vi "GetSetServiceRequestEventMask.vi"(0 "VISA resource name":refnum<visa-resource-name>, 5 "get/set":T1, 7 "Mask bits":u8 step=1, 11 "error in":errorcluster) -> (4 "VISA resource name out":refnum<visa-resource-name>, 6 "SRQ event mask string":string, 8 "SRQ event mask":i32, 10 "SRQ event mask binary":string, 15 "error out":errorcluster)   [LabVIEW 2023, in "Thermotron 8800.lvlib"]
doc: "SRQM\nCommand name: Send or load service request event mask byte\nCommand type: System status\nDescription: This byte enables the various events for requesting service via the GPIB SRQ line. The coded integer data represents the enabled events using the definitions given under the SRQB command.\nNOTE: Setting the SRQ mask to zero disables all SRQ interrupts.\nSyntax: SRQM? or SRQMdata\nData type: Coded integer (0 to 255)\nQuery example: SQRM?\n8800 response: 4 = 00000100 (The end of interval service request bit has been enabled.)\nbit 7 bit 6 bit 5 bit 4 bit 3 bit 2 bit 1 bit 0\n 0 0 0 0 0 1 0 0\nOperation example: SRQM1\n8800 response: 0 (The 8800 loads the SRQ mask with the value 1, enabling the state change SRQ event.)\nbit 7 bit 6 bit 5 bit 4 bit 3 bit 2 bit 1 bit 0\n 0 0 0 0 0 0 0 1"
uses:
  Thermotron 8800.lvlib
  Private/get set.ctl
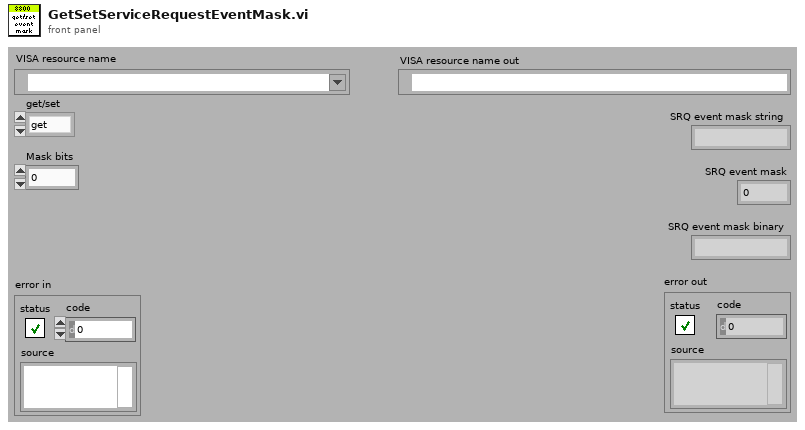
[diagram p1: front panel]
types:
  T1 = typedef "Thermotron 8800.lvlib/get set.ctl" = enum16{"get", "set"}
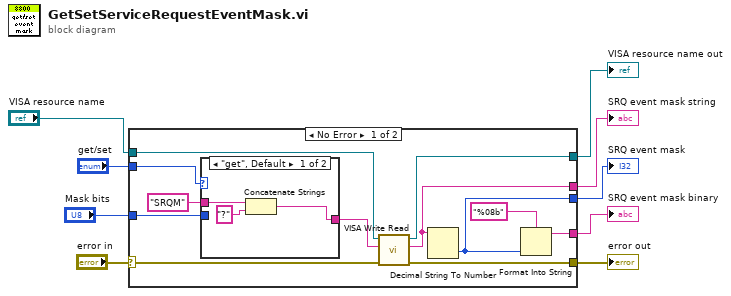
[diagram p0: block diagram]
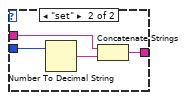
[diagram p2: hidden frame]
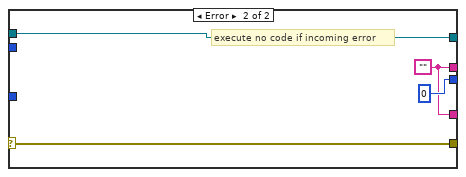
[diagram p3: hidden frame]
diagram:
  n1 = case shown="No Error" "error in" {
    selector: "error in" -> [w14 w31]
    tunnel: "get/set" -> [w21 _]
    tunnel: [w13 w29] -> w3
    tunnel: [w18 w31] -> w6
    tunnel: [w17 w32] -> w8
    tunnel: "VISA resource name" -> [w16 w32]
    tunnel: "Mask bits" -> [w15 _]
    tunnel: [w11 0] -> w2
    tunnel: [w10 w29] -> w1
    frame No Error {
      n2 = case shown="\"get\", Default" w21 {
        tunnel: "SRQM" ("8800 Command") -> [w23 w28]
        tunnel: [w24 w27] -> w19
        tunnel: w15 -> [_ w25]
        frame "get", Default {
          n3 = Concatenate Strings(w23, "?" ("8800 Command")) -> (w24:string)
        }
        frame "set" {
          n4 = Number To Decimal String(number=w25) -> (decimal integer string=w26:string)  [unwired: 1 in]
          n5 = Concatenate Strings(w28, w26) -> (w27:string)
        }
      }
      n6 = call "VISA Write Read.vi"("error in (no error)"=w14, "8800 Command"=w19, "VISA Refnum in"=w16) -> ("error out"=w18:errorcluster, "read buffer"=w13:string, "VISA Refnum out"=w17:refnum<visa-resource-name>)  [unwired: 6 in]
      n7 = Decimal String To Number(string=w13) -> (number=w11:i32)  [unwired: 2 in, 1 out]
      n8 = Format Into String(format string="%08b", w11) -> (resulting string=w10:string)  [unwired: 2 in, 1 out]
    }
    frame Error {
      w29 = ""
      # "execute no code if incoming error"
    }
  }
  "VISA resource name out" <- w8
  "error out" <- w6
  "SRQ event mask string" <- w3
  "SRQ event mask" <- w2
  "SRQ event mask binary" <- w1
